vi "signalWithPeaks.vi"(0 "cutIndex":i32=504000, 1 "filteredECG":dbl[](array[numeric]), 2 "Locations":dbl[](array[numeric]), 3 "# peaks":i32, 4 "batchSize":i32=1500, 5 "lengthOfGraph":i32=2000) -> (7 "2Dsignal/peaks":dbl[][](array[numeric]), 8 "Waveform Graph":dynamicdata(graph))   [LabVIEW 2025]
panel:
  out "Numeric":i32
  out "Numeric 2":i32
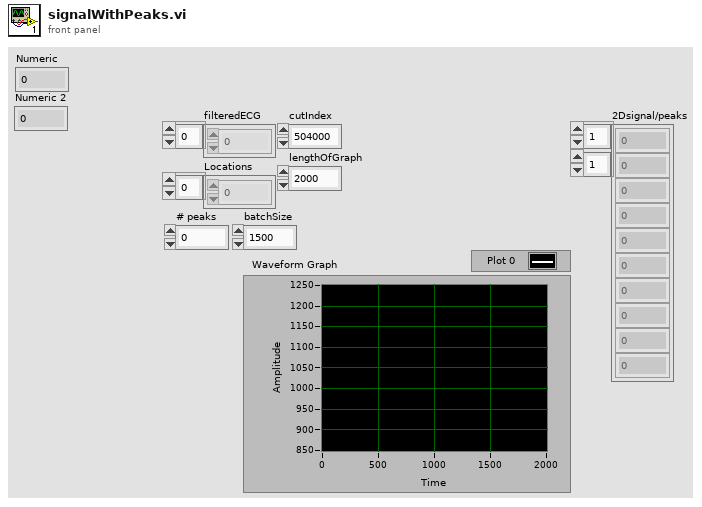
[diagram p1: front panel]
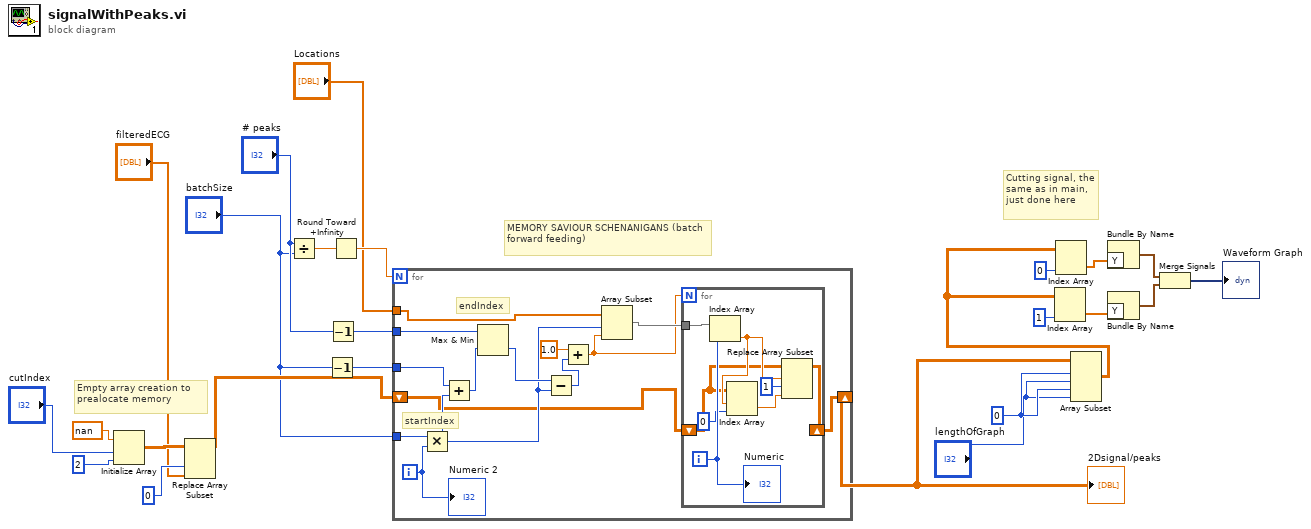
[diagram p0: block diagram]
diagram:
  w17 = 0 ("index")
  # "MEMORY SAVIOUR SCHENANIGANS (batch forward feeding)"
  # "Cutting signal, the same as in main, just done here"
  # "Empty array creation to prealocate memory"
  n1 = Initialize Array(nan ("element"), "cutIndex", 2 ("dimension size")) -> (w23:dbl[][])
  n2 = Replace Array Subset(array=w23, new element="filteredECG", index (col)=0) -> (w8:dbl[][])  [unwired: 1 in]
  n3 = Divide(x="# peaks", y="batchSize") -> (x/y=w21:dbl)
  n4 = Decrement(x="batchSize") -> (x-1=w19:i32)
  n5 = Decrement(x="# peaks") -> (x-1=w18:i32)
  n6 = Round Toward +Infinity(x=w21) -> (ceil(x): smallest int >= x=w20:dbl)
  n7 = for {
    N: w20 -> [_]
    tunnel: "batchSize" -> [w38]
    tunnel: w19 -> [w37]
    tunnel: w18 -> [w35]
    tunnel: "Locations" -> [w34]
    shift-right: [w26] -> w12
    shift-left: w8 -> [w27]
    i -> [w39]
    # "endIndex"
    # "startIndex"
    n8 = Multiply(x=w38, y=w39) -> (x*y=w32:i32)
    n9 = Add(x=w37, y=w32) -> (x+y=w36:i32)
    n10 = Max & Min(x=w35, y=w36) -> (min(x,y)=w33:i32)  [unwired: 1 out]
    n11 = Subtract(x=w33, y=w32) -> (x-y=w31:i32)
    n12 = Add(x=1.0, y=w31) -> (x+y=w28:dbl)
    n13 = Array Subset(array=w34, index=w32, length=w28) -> (w29:dbl[])
    n14 = for {
      N: w28 -> [_]
      tunnel: w29 -> [w47]
      shift-right: [w40] -> w26
      shift-left: w27 -> [w41]
      i -> [w46]
      n15 = Index Array(array=w47, index=w46) -> (element=w44:dbl)
      n16 = Index Array(array=w41, index (row)=w44, index (col)=0) -> (element=w42:dbl)
      n17 = Replace Array Subset(array=w41, new element=w42, index (row)=w44, index (col)=1 ("disabled index (col)")) -> (w40:dbl[][])
      "Numeric" <- w46
    }
    "Numeric 2" <- w39
  }
  "2Dsignal/peaks" <- w12
  n18 = Array Subset(array=w12, index (row)=w17, length (row)="lengthOfGraph", index (col)=w17, length (col)="lengthOfGraph") -> (w11:dbl[][])
  n19 = Index Array(array=w11, index (col)=1 ("disabled index (col)")) -> (element=w13:dbl[])  [unwired: 1 in]
  n20 = Index Array(array=w11, index (col)=0 ("disabled index (col)")) -> (element=w14:dbl[])  [unwired: 1 in]
  n21 = Bundle By Name("Y"=w14) -> (w9:waveform(dbl))  [unwired: 1 in]
  n22 = Bundle By Name("Y"=w13) -> (w10:waveform(dbl))  [unwired: 1 in]
  n23 = Merge Signals(w9, w10) -> (→"Waveform Graph":dynamicdata)
